vi "AuthSrpInitiationResponse_Create.vi"(7 "Header":T3, 8 "error in (no error)":errorcluster, 9 "ResponseError":errorcluster, 10 "AuthSrpInitiationResponse":T1, 11 "IRoutingSource":T2) -> (0 "error out":errorcluster, 3 "Message":T5)   [LabVIEW 2017]
uses:
  <vilib>/addons/InsightCM/MessageBus/Base/controls/Message.ctl
  <vilib>/addons/InsightCM/MessageBus/Base/controls/MessageHeader.ctl
  <vilib>/addons/InsightCM/MessageBus/Base/controls/KeyValuePair.ctl
  <vilib>/addons/InsightCM/MessageBus/Base/controls/IRoutingSource.ctl
  <vilib>/addons/InsightCM/MessageBus/MessageLibrary/Authentication/controls/AuthSrpInitiationResponseBody.ctl
  <vilib>/addons/InsightCM/MessageBus/Base/controls/MessageClassType.ctl
  <vilib>/addons/InsightCM/Utilities/PropertyHelpers/PropertyHelpers.lvlib
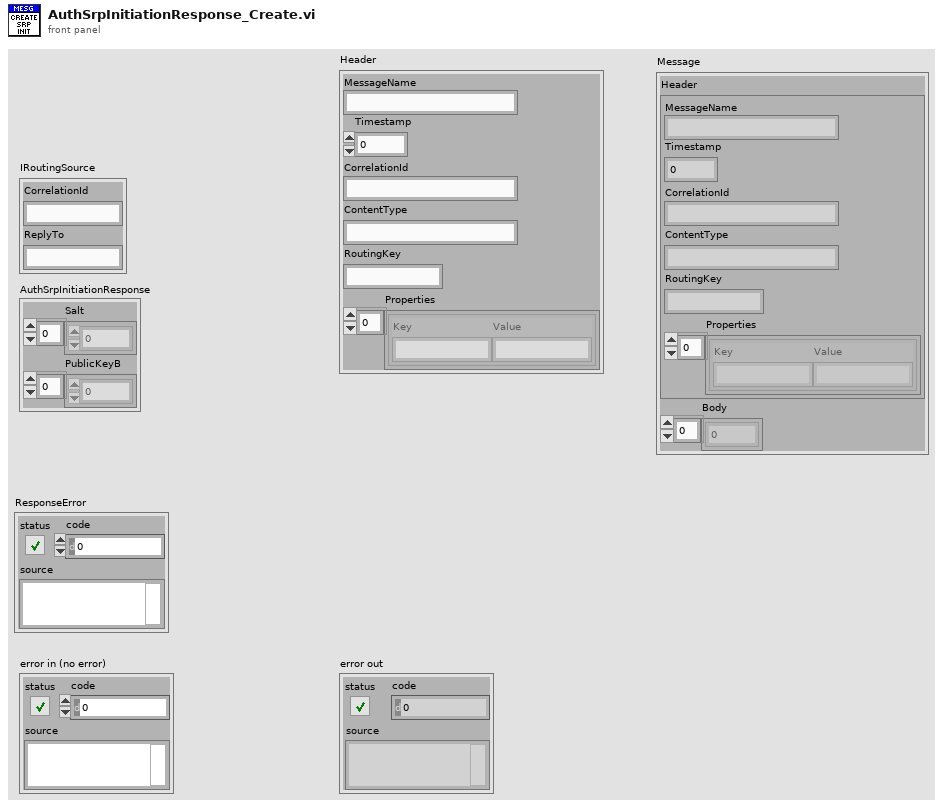
[diagram p1: front panel]
types:
  T1 = typedef "AuthSrpInitiationResponseBody.ctl" = cluster{"Salt":u8[], "PublicKeyB":u8[]}
  T2 = typedef "IRoutingSource.ctl" = cluster{"CorrelationId":string, "ReplyTo":string}
  T3 = typedef "MessageHeader.ctl" = cluster{"MessageName":string, "Timestamp":i64, "CorrelationId":string, "ContentType":string, "RoutingKey":string, "Properties":T4[]}
  T4 = typedef "KeyValuePair.ctl" = cluster{"Key":string, "Value":string}
  T5 = typedef "Message.ctl" = cluster{"Header":T3, "Body":u8[]}
  T6 = typedef "MessageClassType.ctl" = enum16{"Request", "Response", "Broadcast", "RoutedMessage"}
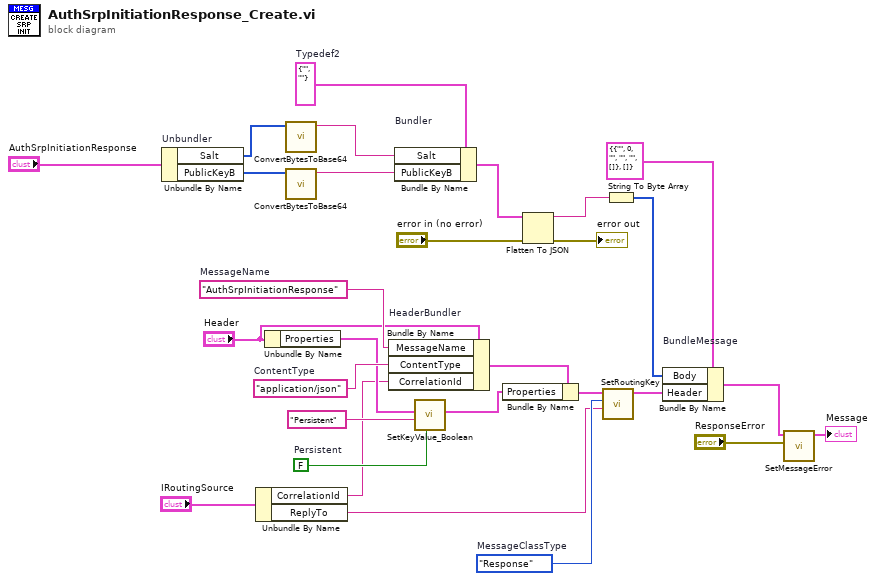
[diagram p0: block diagram]
diagram:
  w5 = cluster{"Salt":string, "PublicKeyB":string} {"Salt"="", "PublicKeyB"=""}  # Typedef2
  w25 = MessageClassType."Response"  # MessageClassType
  w20 = FALSE  # Persistent
  w26 = "AuthSrpInitiationResponse"  # MessageName
  w23 = "application/json"  # ContentType
  n1 = Unbundle By Name "Unbundler"("AuthSrpInitiationResponse") -> ("Salt"=w4:u8[], "PublicKeyB"=w2:u8[])
  n2 = Unbundle By Name("IRoutingSource") -> ("CorrelationId"=w10:string, "ReplyTo"=w9:string)
  n3 = Unbundle By Name("Header") -> ("Properties"=w22:T4[])
  n4 = call <vilib>:"ConvertBytesToBase64.vi"("U8 array"=w4) -> ("base64 encoded"=w3:string)  [unwired: 10 in]
  n5 = call <vilib>:"ConvertBytesToBase64.vi"("U8 array"=w2) -> ("base64 encoded"=w1:string)  [unwired: 10 in]
  n6 = Bundle By Name "HeaderBundler"(cluster="Header", "MessageName"=w26, "ContentType"=w23, "CorrelationId"=w10) -> (w17:T3)
  n7 = Bundle By Name "Bundler"(cluster=w5, "Salt"=w3, "PublicKeyB"=w1) -> (w6:cluster{"Salt":string, "PublicKeyB":string})
  n8 = call <vilib>:"SetKeyValue_Boolean.vi"("value"=w20, "key"="Persistent" ("Key"), "key value pairs"=w22) -> ("key value pairs out"=w16:T4[])  [unwired: 8 in]
  n9 = Bundle By Name(cluster=w17, "Properties"=w16) -> (w18:T3)
  n10 = Flatten To JSON(anything=w6, error in (no error)="error in (no error)") -> (JSON string=w8:string, 11:→"error out":errorcluster)  [unwired: 1 in]
  n11 = call <vilib>:"SetRoutingKey.vi"("SendTo"=w9, "MessageClassType"=w25, "Message Header in"=w18) -> ("Message Header out"=w19:T3)  [unwired: 8 in]
  n12 = String To Byte Array(string=w8) -> (unsigned byte array=w28:u8[])
  n13 = Bundle By Name "BundleMessage"(cluster=T5 {"Header"={"MessageName"="", "Timestamp"=0, "CorrelationId"="", "ContentType"="", "RoutingKey"="", "Properties"=[]}, "Body"=[]} ("Message"), "Body"=w28, "Header"=w19) -> (w14:T5)
  n14 = call <vilib>:"SetMessageError.vi"("error"="ResponseError", "message in"=w14) -> ("message out"=→"Message":T5)  [unwired: 9 in]
